vi "isConnected.vi"(8 "error in (no error)":errorcluster, 11 "Connection in":refnum<class "Connection.lvclass">) -> (0 "error out":errorcluster, 2 "connected":bool, 3 "Connection out":refnum<class "Connection.lvclass">)   [LabVIEW 2013, in "MQTT_Connection.lvlib" / "Connection.lvclass"]
uses:
  Connection.lvclass
  Connection.lvclass/Connection.ctl
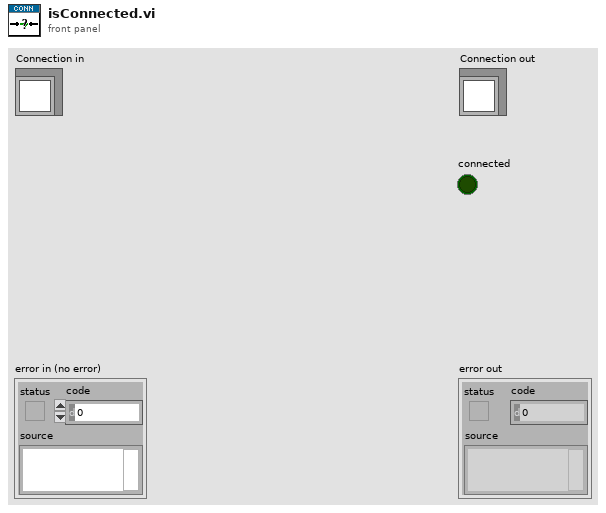
[diagram p1: front panel]
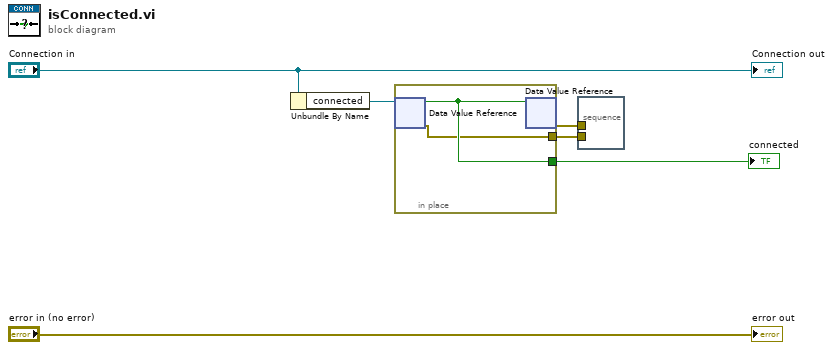
[diagram p0: block diagram]
diagram:
  n1 = Unbundle By Name("Connection in") -> ("connected"=w4:refnum<data-value>)
  n2 = in-place {
    in-place-border: [w8] -> w3
    in-place-border: [w7] -> w1
    n3 = in-place-dvr #1(w4) -> (w8:bool, w7:errorcluster)
    n4 = in-place-dvr #1(w8) -> (w2:errorcluster)  [unwired: 1 out]
  }
  "connected" <- w3
  n5 = stacked-sequence {
    tunnel: w2 -> [_]
    tunnel: w1 -> [_]
    frame #0 {
    }
  }
  "error out" <- "error in (no error)"
  "Connection out" <- "Connection in"
